vi "Local Bus Waveform Test.vi"() -> ()   [LabVIEW 2021]
uses:
  Source/Omni-Bus/Omni_Bus.lvclass
  Source/Omni-Bus/Support/Broad Types.ctl
  Source/Local Bus/Local Bus.lvclass
  <vilib>/Utility/Data Type/Type Definitions/Data Type.ctl
  <vilib>/Utility/Data Type/NI_Data Type.lvlib
  Source/Omni-Bus/Support/Read/Read Waveform.vi
  Source/Omni-Bus/Support/Write/Write Waveform.vi
  <vilib>/measure/NI_MABase.lvlib
  <vilib>/measure/NI_MAPro.lvlib
  C:/Users/Tim/Documents/GitHub/Omni-Bus/Source/Omni-Bus/Bus Access/Bus_Access.lvclass
panel:
  out "Waveform Graph":waveform(dbl)(graph)
  in  "stop":bool
  in  "Tag":string
  out "Tags":string[](array[string])
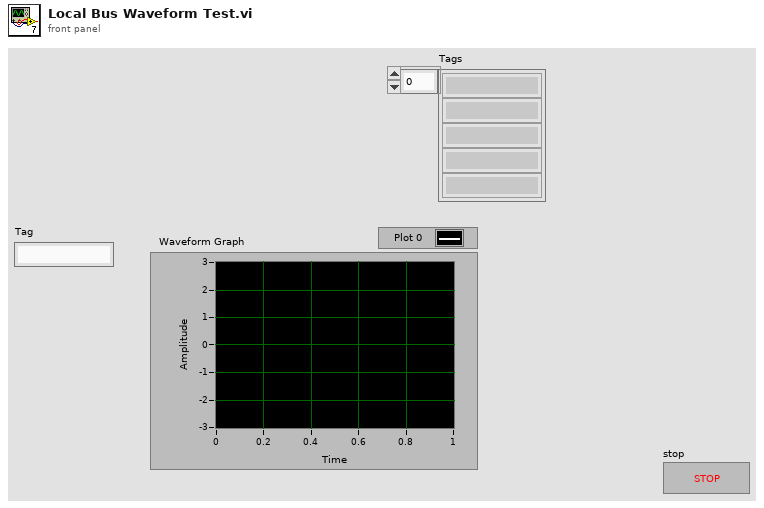
[diagram p1: front panel]
types:
  T1 = typedef "NI_Data Type.lvlib/Data Type.ctl" = enum8{"Invalid Type", "Void", "I8", "I16", "I32", "I64", "U8", "U16", "U32", "U64", "Single Float", "Double Float", "Extended Float", "Single Complex", "Double Complex", "Extended Complex", "Enum U8", "Enum U16", "Enum U32", "Enum U64", "Single Float With Unit", "Double Float With Unit", "Extended Float With Unit", "Single Complex with Unit", "Double Complex with Unit", "Extended Complex with Unit", "Boolean", "String", "Path", "Picture", "Tag", "Array", "Cluster", "Variant", "LV Variant", "Waveform", "Timestamp", "Digital Waveform", "Digital Data", "ExpressData", "Refnum", "External Data", "VI", "Poly VI", "LabVIEW Class Instance", "Fixed Point", "Set Collection", "Map Collection"}
  T2 = typedef "Omni_Bus.lvclass/Broad Types.ctl" = enum16{"All Tags", "NI Specific Type", "Boolean", "String", "Numeric", "Float", "Integer", "Collection", "All Value Types", "Non Value Types"}
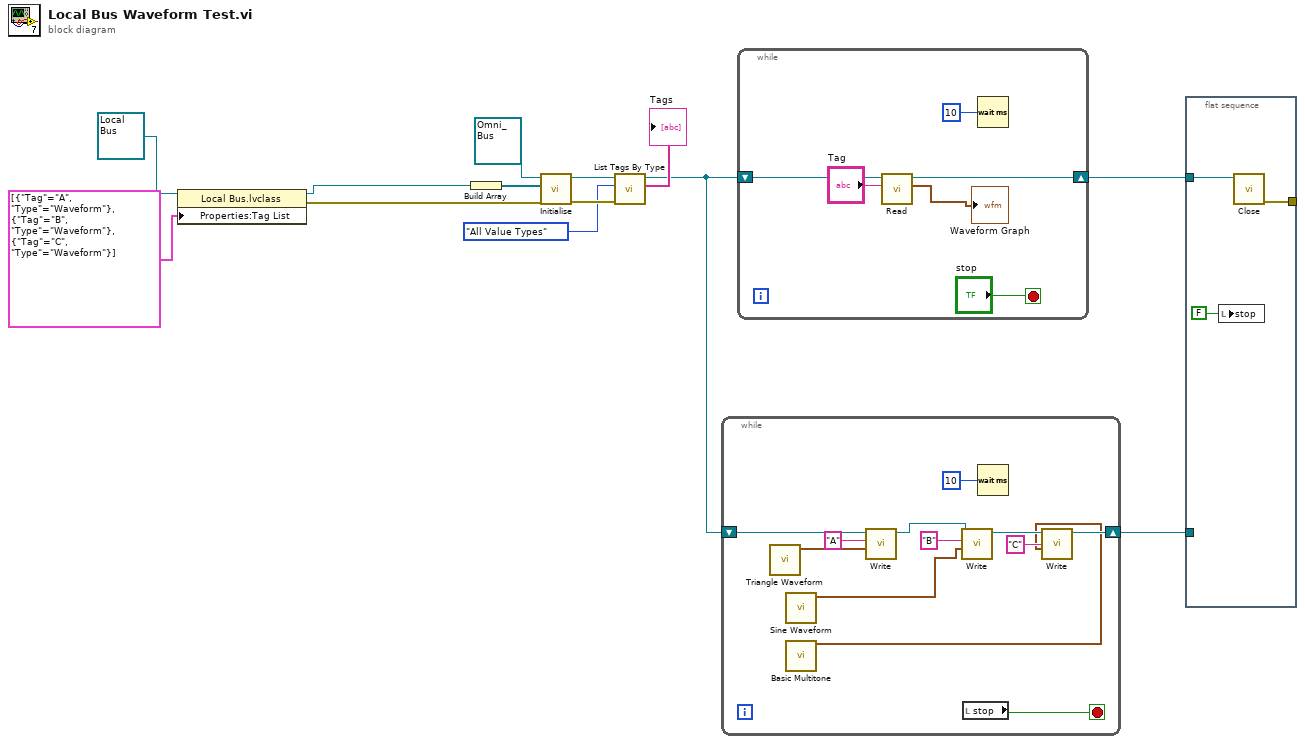
[diagram p0: block diagram]
diagram:
  n1 = property class="Local Bus.lvclass"(reference=refnum<class "Local Bus.lvclass"> refnum ("Local Bus.lvclass"), "Properties:Tag List"=cluster{"Tag":string, "Type":T1}[] [{"Tag"="A", "Type"=enum."Waveform"}, {"Tag"="B", "Type"=enum."Waveform"}, {"Tag"="C", "Type"=enum."Waveform"}] ("Tag List")) -> (reference out=w7:refnum<class "Local Bus.lvclass">, error out=w6:errorcluster)  [unwired: 1 in]
  n2 = Build Array(w7) -> (w12:refnum<class "Local Bus.lvclass">[])
  n3 = call-dynamic "Initialise.vi"("error in (no error)"=w6, "Bus Access"=w12, "Var Bus in"=refnum<class "Omni_Bus.lvclass"> refnum) -> ("error out"=w10:errorcluster, "Var Bus out"=w11:refnum<class "Omni_Bus.lvclass">)  [unwired: 7 in]
  n4 = call-dynamic "List Tags By Type.vi"("error in (no error)"=w10, "Broad Types"=Broad_Types."All Value Types", "Var Bus in"=w11) -> ("Tags"=→"Tags":string[], "Var Bus out"=w2:refnum<class "Omni_Bus.lvclass">)  [unwired: 5 in, 2 out]
  n5 = while {
    shift-right: [w17] -> w1
    shift-left: w2 -> [w25]
    stop <- w24 stop-if-true
    n6 = call <vilib>:"Triangle Waveform.vi"() -> ("signal out"=w14:waveform(dbl))  [unwired: 10 in, 1 out]
    n7 = call <vilib>:"Sine Waveform.vi"() -> ("signal out"=w19:waveform(dbl))  [unwired: 10 in, 1 out]
    n8 = call <vilib>:"Basic Multitone.vi"() -> ("signal out"=w15:waveform(dbl))  [unwired: 12 in, 3 out]
    n9 = call-poly "Write.vi"("Waveform"=w14, "Tag"="A", "Omni_Bus in"=w25) -> ("Omni_Bus out"=w20:refnum<class "Omni_Bus.lvclass">)  [unwired: 7 in, 1 out]
    n10 = call-poly "Write.vi"("Waveform"=w19, "Tag"="B", "Omni_Bus in"=w20) -> ("Omni_Bus out"=w18:refnum<class "Omni_Bus.lvclass">)  [unwired: 7 in, 1 out]
    n11 = local read "stop"() -> (w24:bool)
    n12 = Wait (ms)(milliseconds to wait=u32 10) -> ()  [unwired: 1 out]
    n13 = call-poly "Write.vi"("Waveform"=w15, "Tag"="C", "Omni_Bus in"=w18) -> ("Omni_Bus out"=w17:refnum<class "Omni_Bus.lvclass">)  [unwired: 7 in, 1 out]
  }
  n14 = while {
    shift-right: [w30] -> w3
    shift-left: w2 -> [w31]
    stop <- "stop" stop-if-true
    n15 = call-poly "Read.vi"("Tag"="Tag", "Var Bus in"=w31) -> ("Waveform"=→"Waveform Graph":waveform(dbl), "Var Bus out"=w30:refnum<class "Omni_Bus.lvclass">)  [unwired: 7 in, 1 out]
    n16 = Wait (ms)(milliseconds to wait=u32 10) -> ()  [unwired: 1 out]
  }
  n17 = flat-sequence {
    tunnel: [w34] -> _
    tunnel: w3 -> [w33]
    tunnel: w1 -> [_]
    frame #0 {
      n18 = local write "stop"(FALSE ("stop")) -> ()
      n19 = call-dynamic "Close.vi"("Data in"=w33) -> ("error out"=w34:errorcluster)  [unwired: 9 in, 1 out]
    }
  }
